vi "Frame Read.vi"(8 "error in (no error)":errorcluster caption="entrée d'erreur (pas d'erreur)", 10 "Frame Read":string, 11 "Class Camera  IV3-500CA - Start Program en Entrée":refnum<class "Class Camera  IV3-500CA - Read version.lvclass">) -> (0 "error out":errorcluster caption="sortie d'erreur", 3 "Class Camera  IV3-500CA - Start Program en Sortie":refnum<class "Class Camera  IV3-500CA - Read version.lvclass">)   [LabVIEW 2020, in "Library Instrument & Equipement.lvlib" / "Library Camera.lvlib" / "Class Camera  IV3-500CA - Read version.lvclass"]
uses:
  Class Camera  IV3-500CA - Read version.lvclass
  Class Camera  IV3-500CA - Read version.lvclass/Class Camera  IV3-500CA - Read version.ctl
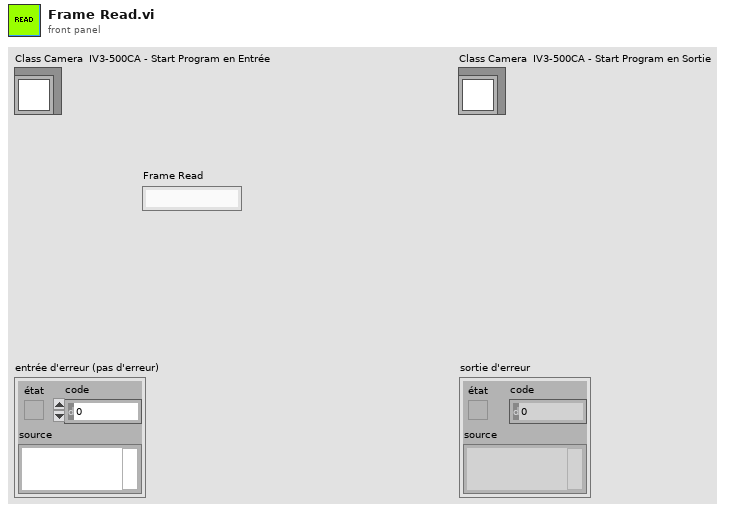
[diagram p1: front panel]
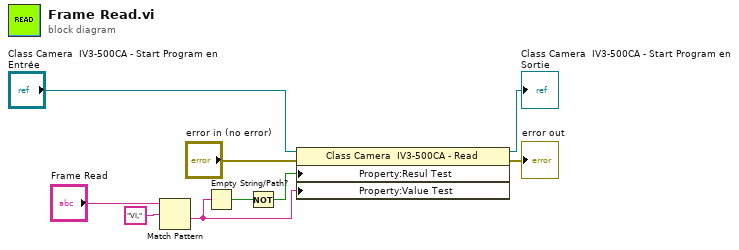
[diagram p0: block diagram]
diagram:
  n1 = Match Pattern(string="Frame Read", regular expression="VI," ("expression régulière")) -> (after substring=w3:string)  [unwired: 1 in, 3 out]
  n2 = Empty String/Path?(string/path=w3) -> (empty?=w2:bool)
  n3 = Not(x=w2) -> (.not. x?=w1:bool)
  n4 = property class="Class Camera  IV3-500CA - Read "(reference="Class Camera  IV3-500CA - Start Program en Entrée", error in="error in (no error)", "Property:Resul Test "=w1, "Property:Value Test"=w3) -> (reference out=→"Class Camera  IV3-500CA - Start Program en Sortie":refnum<class "Class Camera  IV3-500CA - Read version.lvclass">, error out=→"error out":errorcluster)
